vi "Read Digital Port.vi"(0 "Device ID":T2(ring), 5 "Module":T1(ring), 11 "error in":errorcluster) -> (4 "Device ID Out":T2(ring), 6 "Value":bool[](array[boolean]), 15 "error out":errorcluster)   [LabVIEW 2010]
doc: "This VI reads all digital inputs from the transfer area for a given module."
uses:
  Robo Interface.dll
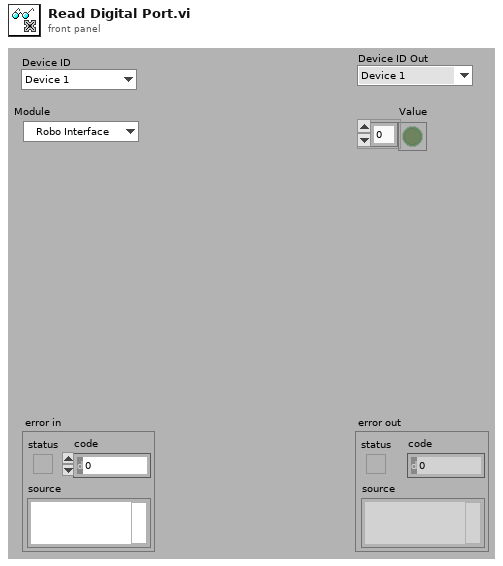
[diagram p1: front panel]
types:
  T1 = enum8{"Robo Interface", "Extension 1", "Extension 2", "Extension 3"}
  T2 = enum16{"Device 1", "Device 2", "Device 3", "Device 4", "Device 5", "Device 6", "Device 7", "Device 8"}
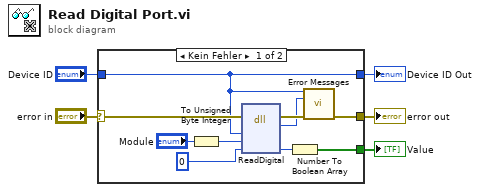
[diagram p0: block diagram]
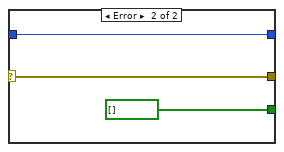
[diagram p2: hidden frame]
diagram:
  n1 = case shown="Kein Fehler" "error in" {
    selector: "error in" -> [w13 w18]
    tunnel: [w12 w18] -> w4
    tunnel: "Device ID" -> [w6 w17]
    tunnel: [w6 w17] -> w2
    tunnel: [w9 bool[] []] -> w1
    frame No Error {
      n2 = To Unsigned Byte Integer(number="Module") -> (unsigned 8bit integer=w14:u8)
      n3 = dll-call lib="D:/Aron/LabVIEW-Programmierung/a.F.b.u.s.A/robo_interface_distribute/Robo Interface/Advanced/Robo Interface.dll" fn="ReadDigital"(error in=w13, "Device_ID"=w6, "Module"=w14, "Value"=u8 0 ("unsigned 8bit integer")) -> (error out=w10:errorcluster, "return type"=w7:i32, "Value"=w11:u8)  [unwired: 3 in, 2 out]
      n4 = Number To Boolean Array(number=w11) -> (Boolean array=w9:bool[])
      n5 = call "Error Messages.vi"("Device ID"=w6, "Error Code"=w7, "error in (no error)"=w10) -> ("error out"=w12:errorcluster)  [unwired: 12 out]
    }
    frame Error {
    }
  }
  "error out" <- w4
  "Device ID Out" <- w2
  "Value" <- w1
